vi "Unit Address.vi"(6 "Settle (1mS)":u32=1, 7 "Address (6)":i16=6, 8 "error in (no error)":errorcluster, 10 "Language Selector (-1)":i16(ring)=-1 items=["none"=-1, "GEN"=0, "SCPI"=1], 11 "VISA resource name":refnum<visa-resource-name>) -> (0 "error out":errorcluster, 3 "VISA resource name out":refnum<visa-resource-name>)   [LabVIEW 2012, in "TDK-Lambda Z.lvlib"]
doc: "Apply to selected address and disconnect previously connected unit"
uses:
  TDK-Lambda Z.lvlib
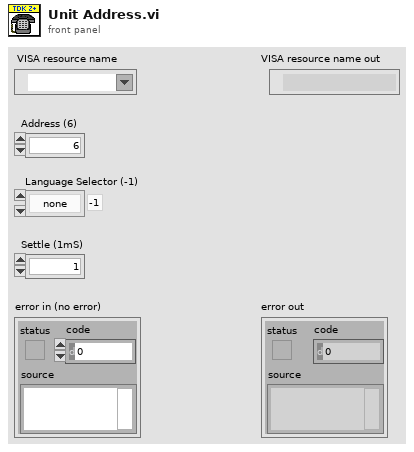
[diagram p1: front panel]
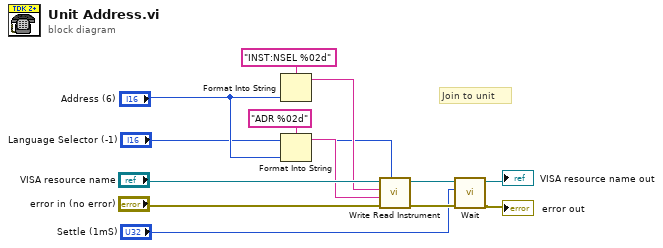
[diagram p0: block diagram]
diagram:
  # "Join to unit"
  n1 = Format Into String(format string="INST:NSEL %02d", "Address (6)") -> (resulting string=w3:string)  [unwired: 2 in, 1 out]
  n2 = Format Into String(format string="ADR %02d", "Address (6)") -> (resulting string=w4:string)  [unwired: 2 in, 1 out]
  n3 = call "Write Read Instrument.vi"("Language Selector (-1)"="Language Selector (-1)", "error in (no error)"="error in (no error)", "GEN  Write Command/Query"=w4, "SCPI  Write Command/Query"=w3, "VISA resource name"="VISA resource name") -> ("error out"=w10:errorcluster, "VISA resource name out"=w11:refnum<visa-resource-name>)  [unwired: 4 in, 1 out]
  n4 = call "Wait.vi"("error in (no error)"=w10, "Wait (1mS)"="Settle (1mS)", "VISA resource name"=w11) -> ("error out"=→"error out":errorcluster, "VISA resource name out"=→"VISA resource name out":refnum<visa-resource-name>)  [unwired: 7 in]
